vi "SwerveModuleOdometry.vi"(6 "Robot Heading(deg)":dbl, 9 "Swerve Encoder Data":T1) -> (0 "Delta Y (in)":dbl, 1 "Delta X (in)":dbl, 2 "Velocity Y (ft/s)":dbl, 3 "Velocity X (ft/s)":dbl)   [LabVIEW 2023]
doc: "This VI calculates the field-centric delta odometry and velocity vectors for a single swerve module."
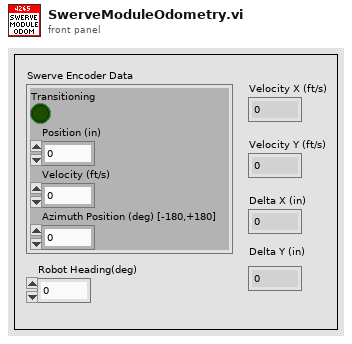
[diagram p1: front panel]
types:
  T1 = cluster{"Transitioning":bool, "Position (in)":dbl, "Velocity (ft/s)":dbl, "Azimuth Position (deg) [-180,+180]":dbl}
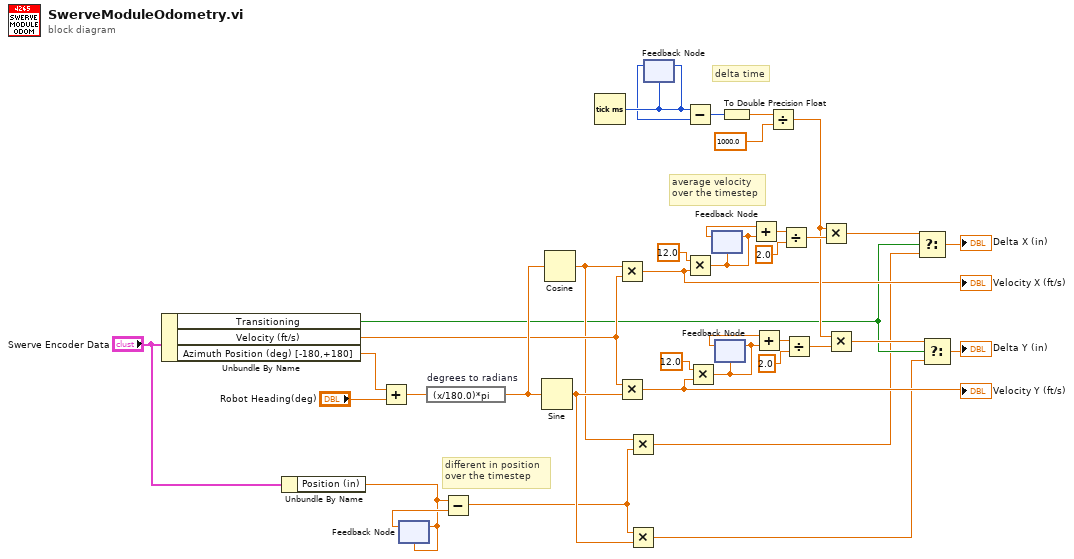
[diagram p0: block diagram]
diagram:
  # "different in position\nover the timestep"
  # "delta time"
  # "average velocity\nover the timestep"
  n1 = Unbundle By Name("Swerve Encoder Data") -> ("Transitioning"=w5:bool, "Velocity (ft/s)"=w17:dbl, "Azimuth Position (deg) [-180,+180]"=w16:dbl)
  n2 = Unbundle By Name("Swerve Encoder Data") -> ("Position (in)"=w2:dbl)
  n3 = Add(x=w16, y="Robot Heading(deg)") -> (x+y=w37:dbl)
  n4 = feedback #1(w2) -> (w12:dbl)
  n5 = feedback-in #1(w2) -> ()
  n6 = expression code="(x/180.0)*pi" "degrees to radians"(w37) -> (w31:dbl)
  n7 = Subtract(x=w2, y=w12) -> (x-y=w1:dbl)
  n8 = Sine(x=w31) -> (sin(x)=w14:dbl)
  n9 = Cosine(x=w31) -> (cos(x)=w13:dbl)
  n10 = Tick Count (ms)() -> (millisecond timer value=w36:u32)
  n11 = Multiply(x=w13, y=w17) -> (x*y=w7:dbl)
  "Velocity X (ft/s)" <- w7
  n12 = Multiply(x=w17, y=w14) -> (x*y=w6:dbl)
  "Velocity Y (ft/s)" <- w6
  n13 = Multiply(x=w13, y=w1) -> (x*y=w4:dbl)
  n14 = Multiply(x=w1, y=w14) -> (x*y=w3:dbl)
  n15 = feedback-in #2(w36) -> ()
  n16 = feedback #2(w36) -> (w35:u32)
  n17 = Subtract(x=w36, y=w35) -> (x-y=w34:u32)
  n18 = Multiply(x=12.0 ("y"), y=w7) -> (x*y=w27:dbl)
  n19 = Multiply(x=12.0 ("y"), y=w6) -> (x*y=w22:dbl)
  n20 = feedback #3(w27) -> (w26:dbl)
  n21 = feedback-in #3(w27) -> ()
  n22 = feedback #4(w22) -> (w21:dbl)
  n23 = feedback-in #4(w22) -> ()
  n24 = To Double Precision Float(number=w34) -> (double precision float=w33:dbl)
  n25 = Add(x=w26, y=w27) -> (x+y=w29:dbl)
  n26 = Add(x=w21, y=w22) -> (x+y=w24:dbl)
  n27 = Divide(x=w33, y=1000.0) -> (x/y=w18:dbl)
  n28 = Divide(x=w29, y=2.0) -> (x/y=w20:dbl)
  n29 = Divide(x=w24, y=2.0) -> (x/y=w19:dbl)
  n30 = Multiply(x=w18, y=w20) -> (x*y=w9:dbl)
  n31 = Multiply(x=w18, y=w19) -> (x*y=w8:dbl)
  n32 = Select(t=w9, s=w5, f=w4) -> (s? t:f=→"Delta X (in)":dbl)
  n33 = Select(t=w8, s=w5, f=w3) -> (s? t:f=→"Delta Y (in)":dbl)
